vi "TEST Config Unicode.vi"() -> ()   [LabVIEW 2013, in "Carya Config.lvclass"]
doc: "Copyright 2018, Carya Automatisering, Wiebe Walstra."
uses:
  Carya Config.lvclass
  CConfig Encoding/CConfig UCS-16 Encoding/CConfig UCS-16 Encoding.lvclass
panel:
  out "Array":bool[](array[boolean])
  out "Original copy":string[](array[string])
  out "Array 2":string[](array[string])
  out "UTF-8":string[](array[string])
  out "Original":string[](array[string])
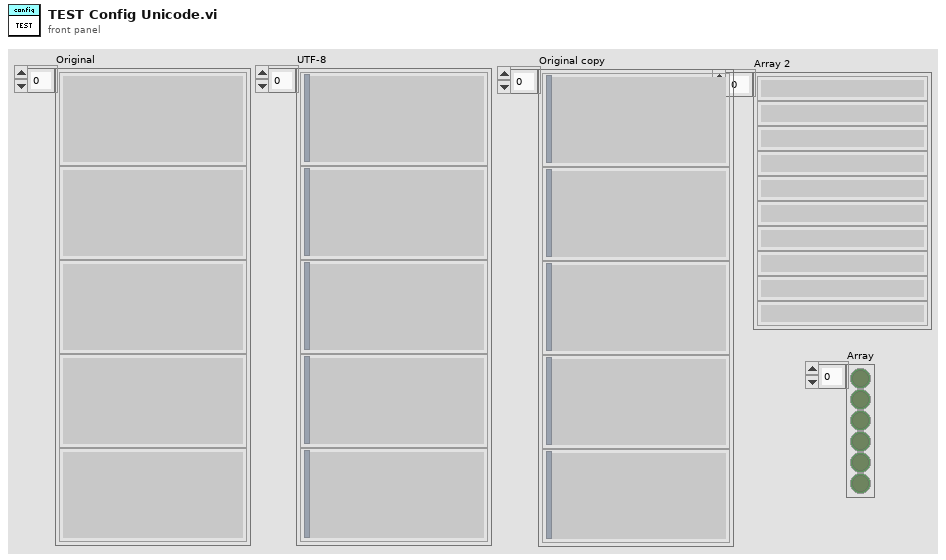
[diagram p1: front panel]
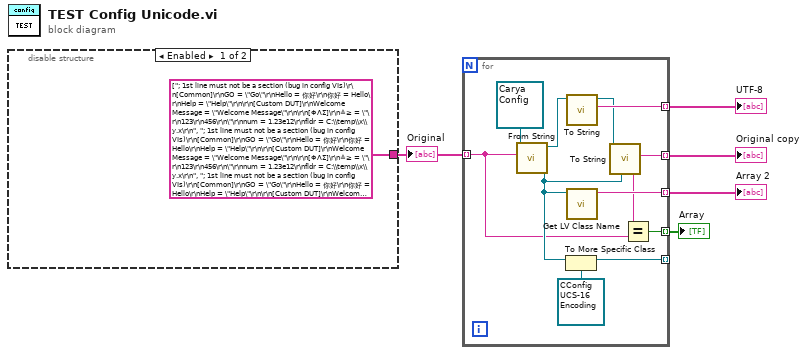
[diagram p0: block diagram]
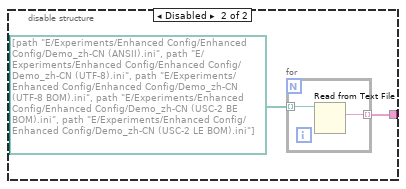
[diagram p2: hidden frame]
diagram:
  n1 = disable-structure shown="Enabled" {
    disable-tunnel: [string[] ["; 1st line must not be a section (bug in config VIs)\r\n[Common]\r\nGO = \"Go\"\r\nHello = 你好\r\n你好 = Hello\r\nHelp = \"Help\"\r\n\r\n[Custom DUT]\r\nWelcome Message = \"Welcome Message\"\r\n\r\n[ΦΛΣ]\r\n≗≥ = \"\r\n123\r\n456\r\n\"\r\nnum = 1.23e12\r\nfldr = C:\\temp\\x\\y.x\r\n", "; 1st line must not be a section (bug in config VIs)\r\n[Common]\r\nGO = \"Go\"\r\nHello = 你好\r\n你好 = Hello\r\nHelp = \"Help\"\r\n\r\n[Custom DUT]\r\nWelcome Message = \"Welcome Message\"\r\n\r\n[ΦΛΣ]\r\n≗≥ = \"\r\n123\r\n456\r\n\"\r\nnum = 1.23e12\r\nfldr = C:\\temp\\x\\y.x\r\n", "﻿; 1st line must not be a section (bug in config VIs)\r\n[Common]\r\nGO = \"Go\"\r\nHello = 你好\r\n你好 = Hello\r\nHelp = \"Help\"\r\n\r\n[Custom DUT]\r\nWelcome Message = \"Welcome Message\"\r\n\r\n[ΦΛΣ]\r\n≗≥ = \"\r\n123\r\n456\r\n\"\r\nnum = 1.23e12\r\nfldr = C:\\temp\\x\\y.x\r\n", "þÿ\u0000;\u0000 \u00001\u0000s\u0000t\u0000 \u0000l\u0000i\u0000n\u0000e\u0000 \u0000m\u0000u\u0000s\u0000t\u0000 \u0000n\u0000o\u0000t\u0000 \u0000b\u0000e\u0000 \u0000a\u0000 \u0000s\u0000e\u0000c\u0000t\u0000i\u0000o\u0000n\u0000 \u0000(\u0000b\u0000u\u0000g\u0000 \u0000i\u0000n\u0000 \u0000c\u0000o\u0000n\u0000f\u0000i\u0000g\u0000 \u0000V\u0000I\u0000s\u0000)\u0000\r\u0000\n\u0000[\u0000C\u0000o\u0000m\u0000m\u0000o\u0000n\u0000]\u0000\r\u0000\n\u0000G\u0000O\u0000 \u0000=\u0000 \u0000\"\u0000G\u0000o\u0000\"\u0000\r\u0000\n\u0000H\u0000e\u0000l\u0000l\u0000o\u0000 \u0000=\u0000 O`Y}\u0000\r\u0000\nO`Y}\u0000 \u0000=\u0000 \u0000H\u0000e\u0000l\u0000l\u0000o\u0000\r\u0000\n\u0000H\u0000e\u0000l\u0000p\u0000 \u0000=\u0000 \u0000\"\u0000H\u0000e\u0000l\u0000p\u0000\"\u0000\r\u0000\n\u0000\r\u0000\n\u0000[\u0000C\u0000u\u0000s\u0000t\u0000o\u0000m\u0000 \u0000D\u0000U\u0000T\u0000]\u0000\r\u0000\n\u0000W\u0000e\u0000l\u0000c\u0000o\u0000m\u0000e\u0000 \u0000M\u0000e\u0000s\u0000s\u0000a\u0000g\u0000e\u0000 \u0000=\u0000 \u0000\"\u0000W\u0000e\u0000l\u0000c\u0000o\u0000m\u0000e\u0000 \u0000M\u0000e\u0000s\u0000s\u0000a\u0000g\u0000e\u0000\"\u0000\r\u0000\n\u0000\r\u0000\n\u0000[\u0003¦\u0003›\u0003£\u0000]\u0000\r\u0000\n\"W\"e\u0000 \u0000=\u0000 \u0000\"\u0000\r\u0000\n\u00001\u00002\u00003\u0000\r\u0000\n\u00004\u00005\u00006\u0000\r\u0000\n\u0000\"\u0000\r\u0000\n\u0000n\u0000u\u0000m\u0000 \u0000=\u0000 \u00001\u0000.\u00002\u00003\u0000e\u00001\u00002\u0000\r\u0000\n\u0000f\u0000l\u0000d\u0000r\u0000 \u0000=\u0000 \u0000C\u0000:\u0000\\\u0000t\u0000e\u0000m\u0000p\u0000\\\u0000x\u0000\\\u0000y\u0000.\u0000x\u0000\r\u0000\n", "ÿþ;\u0000 \u00001\u0000s\u0000t\u0000 \u0000l\u0000i\u0000n\u0000e\u0000 \u0000m\u0000u\u0000s\u0000t\u0000 \u0000n\u0000o\u0000t\u0000 \u0000b\u0000e\u0000 \u0000a\u0000 \u0000s\u0000e\u0000c\u0000t\u0000i\u0000o\u0000n\u0000 \u0000(\u0000b\u0000u\u0000g\u0000 \u0000i\u0000n\u0000 \u0000c\u0000o\u0000n\u0000f\u0000i\u0000g\u0000 \u0000V\u0000I\u0000s\u0000)\u0000\r\u0000\n\u0000[\u0000C\u0000o\u0000m\u0000m\u0000o\u0000n\u0000]\u0000\r\u0000\n\u0000G\u0000O\u0000 \u0000=\u0000 \u0000\"\u0000G\u0000o\u0000\"\u0000\r\u0000\n\u0000H\u0000e\u0000l\u0000l\u0000o\u0000 \u0000=\u0000 \u0000`O}Y\r\u0000\n\u0000`O}Y \u0000=\u0000 \u0000H\u0000e\u0000l\u0000l\u0000o\u0000\r\u0000\n\u0000H\u0000e\u0000l\u0000p\u0000 \u0000=\u0000 \u0000\"\u0000H\u0000e\u0000l\u0000p\u0000\"\u0000\r\u0000\n\u0000\r\u0000\n\u0000[\u0000C\u0000u\u0000s\u0000t\u0000o\u0000m\u0000 \u0000D\u0000U\u0000T\u0000]\u0000\r\u0000\n\u0000W\u0000e\u0000l\u0000c\u0000o\u0000m\u0000e\u0000 \u0000M\u0000e\u0000s\u0000s\u0000a\u0000g\u0000e\u0000 \u0000=\u0000 \u0000\"\u0000W\u0000e\u0000l\u0000c\u0000o\u0000m\u0000e\u0000 \u0000M\u0000e\u0000s\u0000s\u0000a\u0000g\u0000e\u0000\"\u0000\r\u0000\n\u0000\r\u0000\n\u0000[\u0000¦\u0003›\u0003£\u0003]\u0000\r\u0000\n\u0000W\"e\" \u0000=\u0000 \u0000\"\u0000\r\u0000\n\u00001\u00002\u00003\u0000\r\u0000\n\u00004\u00005\u00006\u0000\r\u0000\n\u0000\"\u0000\r\u0000\n\u0000n\u0000u\u0000m\u0000 \u0000=\u0000 \u00001\u0000.\u00002\u00003\u0000e\u00001\u00002\u0000\r\u0000\n\u0000f\u0000l\u0000d\u0000r\u0000 \u0000=\u0000 \u0000C\u0000:\u0000\\\u0000t\u0000e\u0000m\u0000p\u0000\\\u0000x\u0000\\\u0000y\u0000.\u0000x\u0000\r\u0000\n\u0000"] ("Array 4") w7] -> w3
    frame Enabled {
    }
    frame Disabled {
      n2 = for {
        tunnel: path[] [path "E:/Experiments/Enhanced Config/Enhanced Config/Demo_zh-CN (ANSII).ini", path "E:/Experiments/Enhanced Config/Enhanced Config/Demo_zh-CN (UTF-8).ini", path "E:/Experiments/Enhanced Config/Enhanced Config/Demo_zh-CN (UTF-8 BOM).ini", path "E:/Experiments/Enhanced Config/Enhanced Config/Demo_zh-CN (USC-2 BE BOM).ini", path "E:/Experiments/Enhanced Config/Enhanced Config/Demo_zh-CN (USC-2 LE BOM).ini"] -> [w10] mode=indexing
        tunnel: [w9] -> w7 mode=indexing
        n3 = Read from Text File(file (use dialog)=w10) -> (text=w9:string)  [unwired: 3 in, 3 out]
      }
    }
  }
  "Original" <- w3
  n4 = for {
    tunnel: w3 -> [w12] mode=indexing
    tunnel: [w19] -> w5 mode=indexing
    tunnel: [w18] -> w4 mode=indexing
    tunnel: [w16] -> _ mode=indexing
    tunnel: [w13] -> w2 mode=indexing
    tunnel: [w11] -> w1 mode=indexing
    n5 = call-dynamic "From String.vi"("String"=w12, "Carya Config in"=refnum<class "Carya Config.lvclass"> refnum) -> ("Used encoding"=w14:refnum<class "CConfig Encoding.lvclass">, "Carya Config out"=w20:refnum<class "Carya Config.lvclass">)  [unwired: 7 in, 1 out]
    n6 = To More Specific Class(target class=refnum<class "CConfig UCS-16 Encoding.lvclass"> refnum ("CConfig UCS-16 Encoding.lvclass"), reference=w14) -> (specific class reference=w16:refnum<class "CConfig UCS-16 Encoding.lvclass">)  [unwired: 1 in, 1 out]
    n7 = call-dynamic "To String.vi"("Carya Config in"=w20) -> ("String"=w19:string, "Carya Config out"=w15:refnum<class "Carya Config.lvclass">)  [unwired: 8 in, 1 out]
    n8 = call <vilib>:"Get LV Class Name.vi"("object"=w14) -> ("class name"=w18:string)  [unwired: 9 in, 1 out]
    n9 = call-dynamic "To String.vi"("Encoding [No encoding]"=w14, "Carya Config in"=w15) -> ("String"=w13:string)  [unwired: 7 in, 2 out]
    n10 = Equal?(x=w13, y=w12) -> (x = y?=w11:bool)
  }
  "UTF-8" <- w5
  "Array 2" <- w4
  "Original copy" <- w2
  "Array" <- w1
